vi "CREATE TABLE.vi"(8 "error in":errorcluster, 10 "cols & types":string, 11 "ORM Scripter in":refnum<class "ORM Scripter.lvclass">) -> (0 "error out":errorcluster, 1 "create script":string, 3 "ORM Scripter out":refnum<class "ORM Scripter.lvclass">)   [LabVIEW 2018, in "ORM Scripter.lvclass"]
uses:
  ORM Scripter.lvclass
  ORM Scripter.lvclass/ORM Scripter.ctl
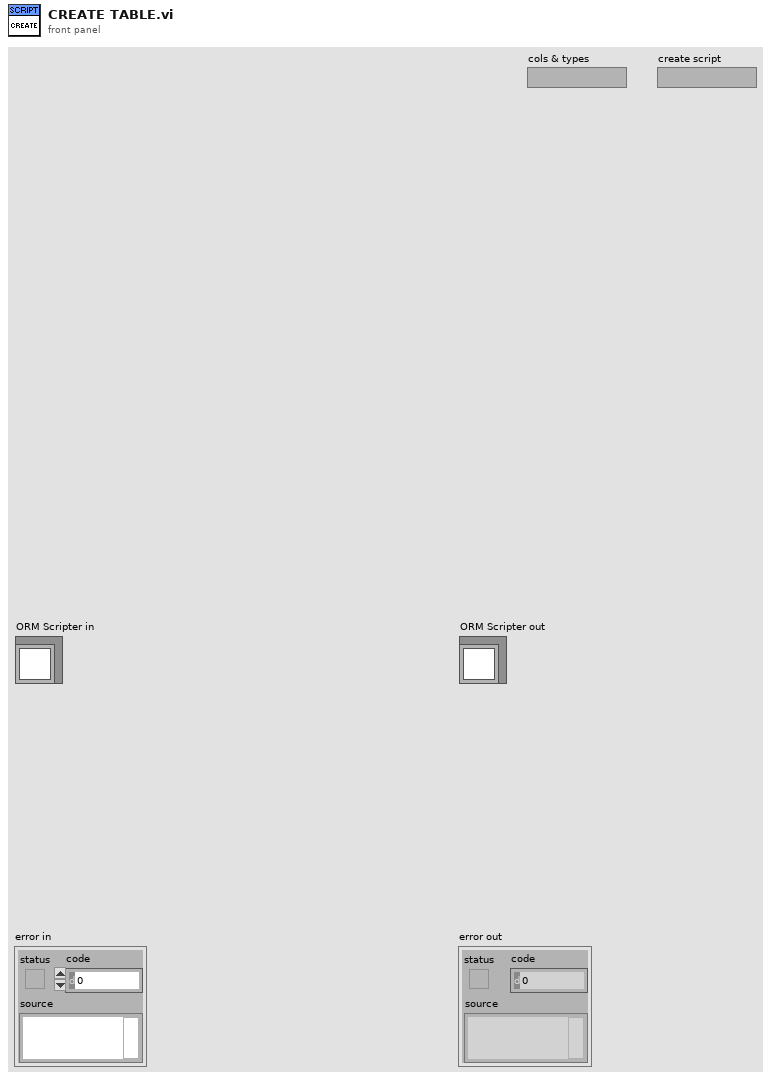
[diagram p1: front panel]
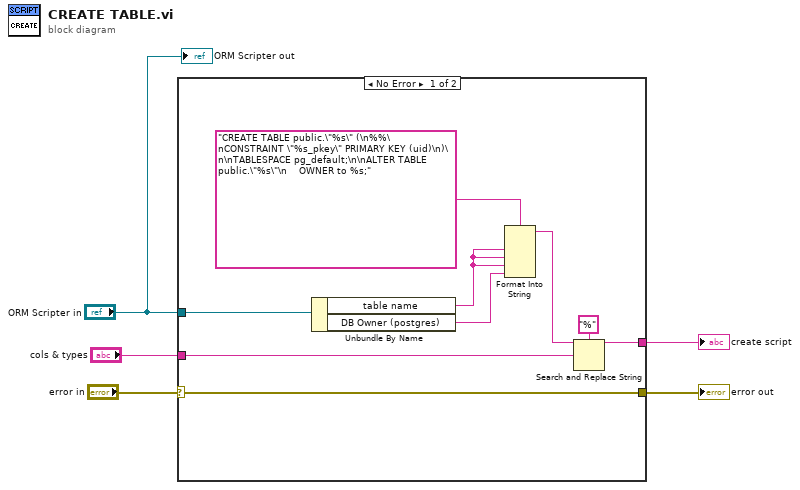
[diagram p0: block diagram]
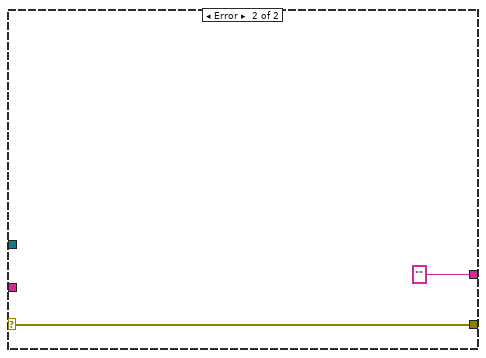
[diagram p2: hidden frame]
diagram:
  n1 = case shown="No Error" "error in" {
    selector: "error in" -> [w6 w15]
    tunnel: "cols & types" -> [w14 _]
    tunnel: [w13 ""] -> w4
    tunnel: "ORM Scripter in" -> [w10 _]
    tunnel: [w6 w15] -> w1
    frame No Error {
      n2 = Unbundle By Name(w10) -> ("table name"=w9:string, "DB Owner (postgres)"=w8:string)
      n3 = Format Into String(format string="CREATE TABLE public.\"%s\" (\n%%\nCONSTRAINT \"%s_pkey\" PRIMARY KEY (uid)\n)\n\nTABLESPACE pg_default;\n\nALTER TABLE public.\"%s\"\n    OWNER to %s;", w9, w9, w9, w8) -> (resulting string=w7:string)  [unwired: 2 in, 1 out]
      n4 = Search and Replace String(input string=w7, search string="%", replace string=w14) -> (result string=w13:string)  [unwired: 5 in, 3 out]
    }
    frame Error {
    }
  }
  "create script" <- w4
  "error out" <- w1
  "ORM Scripter out" <- "ORM Scripter in"
